vi "RgbaToU64_1D.vi"(11 "Rgba":T1[](array[typedef])) -> (3 "U64":u64[](array[numeric]))   [LabVIEW 2020, in "OpenLvVision_Image.lvlib" / "DataAccess.lvlib"]
doc: "Convert an color cluster into an number"
uses:
  DataAccess.lvlib
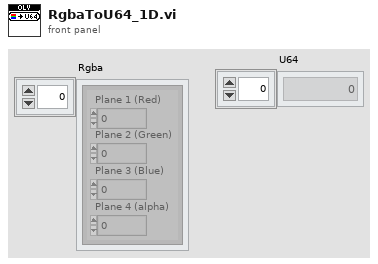
[diagram p1: front panel]
types:
  T1 = typedef "Color (U64)" = cluster{"Plane 3 (Blue)":u16, "Plane 2 (Green)":u16, "Plane 1 (Red)":u16, "Plane 4 (alpha)":u16}
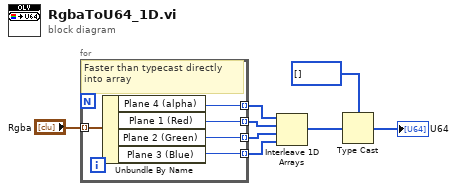
[diagram p0: block diagram]
diagram:
  n1 = for {
    tunnel: "Rgba" -> [w13] mode=indexing
    tunnel: [w12] -> w8 mode=indexing
    tunnel: [w11] -> w6 mode=indexing
    tunnel: [w10] -> w7 mode=indexing
    tunnel: [w9] -> w5 mode=indexing
    # "Faster than typecast directly into array"
    n2 = Unbundle By Name(w13) -> ("Plane 4 (alpha)"=w12:u16, "Plane 1 (Red)"=w11:u16, "Plane 2 (Green)"=w10:u16, "Plane 3 (Blue)"=w9:u16)
  }
  n3 = Interleave 1D Arrays(w8, w6, w7, w5) -> (w4:u16[])
  n4 = Type Cast(type=u64[] [], x=w4) -> (*(type *) &x=→"U64":u64[])
